vi "Durability_will_2012_07_09.vi"() -> ()   [LabVIEW 2011]
uses:
  <vilib>/DAQmx/read.llb/DAQmx Read (Analog 1D Wfm NChan NSamp).vi
  <vilib>/DAQmx/write.llb/DAQmx Write (Counter Time 1Chan 1Samp).vi
  <vilib>/measure/madcrms.llb/Basic Averaged DC-RMS for 1 Chan.vi
  <vilib>/DAQmx/miscellaneous.llb/DAQmx Fill In Error Info.vi
  <vilib>/Analysis/NI_AALBase.lvlib
  <vilib>/measure/NI_MAPro.lvlib
panel:
  in  "Motor1 ID":string
  in  "User":string
  in  "Comments (cleared when written to file)":string
  out "Motor 1 Elapsed Time (s)":string caption="Elapsed Time Text"
  out "Motor 1 Start Time":string caption="Start Time Text"
  out "Motor 1 Down":bool
  out "Long Write":bool caption="Time has Elapsed"
  out "Short Write":bool caption="Time has Elapsed"
  out "Temps":dynamicdata(graph) caption="Signal Out"
  out "Power Graph":dynamicdata(graph) caption="Collected Signals"
  out "Errors":errorcluster
  out "RPM":dynamicdata(graph) caption="Collected Signals"
  out "Motor RPM":dbl format="%#.0f"
  out "Motor Power (watts)":dbl format="%#.4f"
  out "Power to MC1 (watts)":dbl format="%#.4f"
  out "Voltage to MC1 (volts)":dbl format="%#.4f"
  out "Current to MC1  (amps)":dbl format="%#.4f"
  in  "Manual Start":bool
  in  "Power \nSetting":i8(slide) min=0 max=100 step=10 scale=0.0..100.0
  out "Motor Temp (F)":dbl format="%.1f"
  out "Tank Temp (F)":dbl format="%.1f"
  in  "Quit 4":bool
  out "Phase to Phase Voltage":waveform(dbl)(graph)
  out "Phase Current":waveform(dbl)(graph)
  # "Temperature"
  # "MC1"
  # "Motor Power and RPM"
  # "todo disable user and motor fields when file started writing"
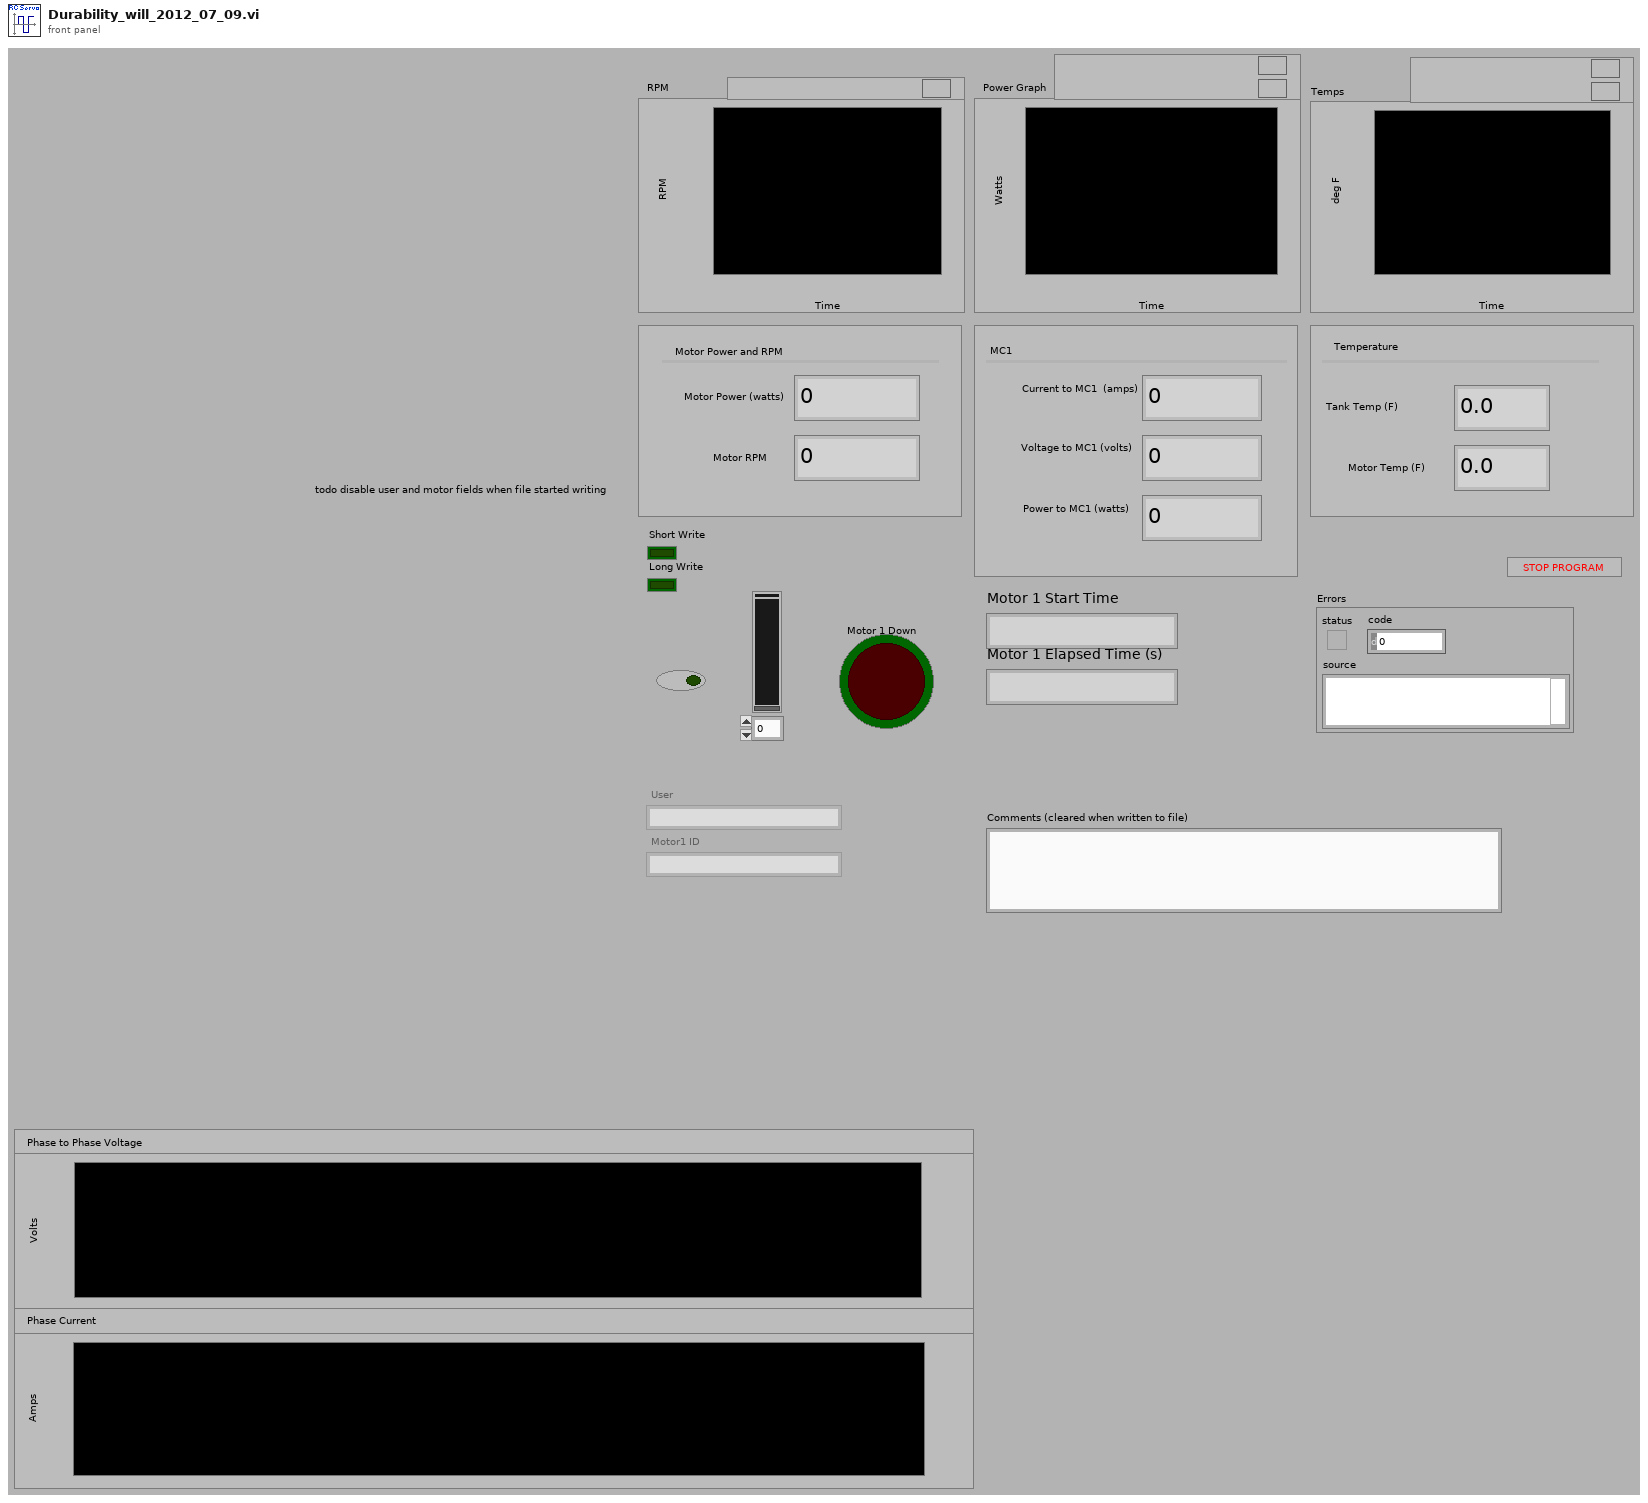
[diagram p1: front panel]
types:
  T1 = enum8{"Enabled", "Disabled", "Disabled and Grayed Out"}
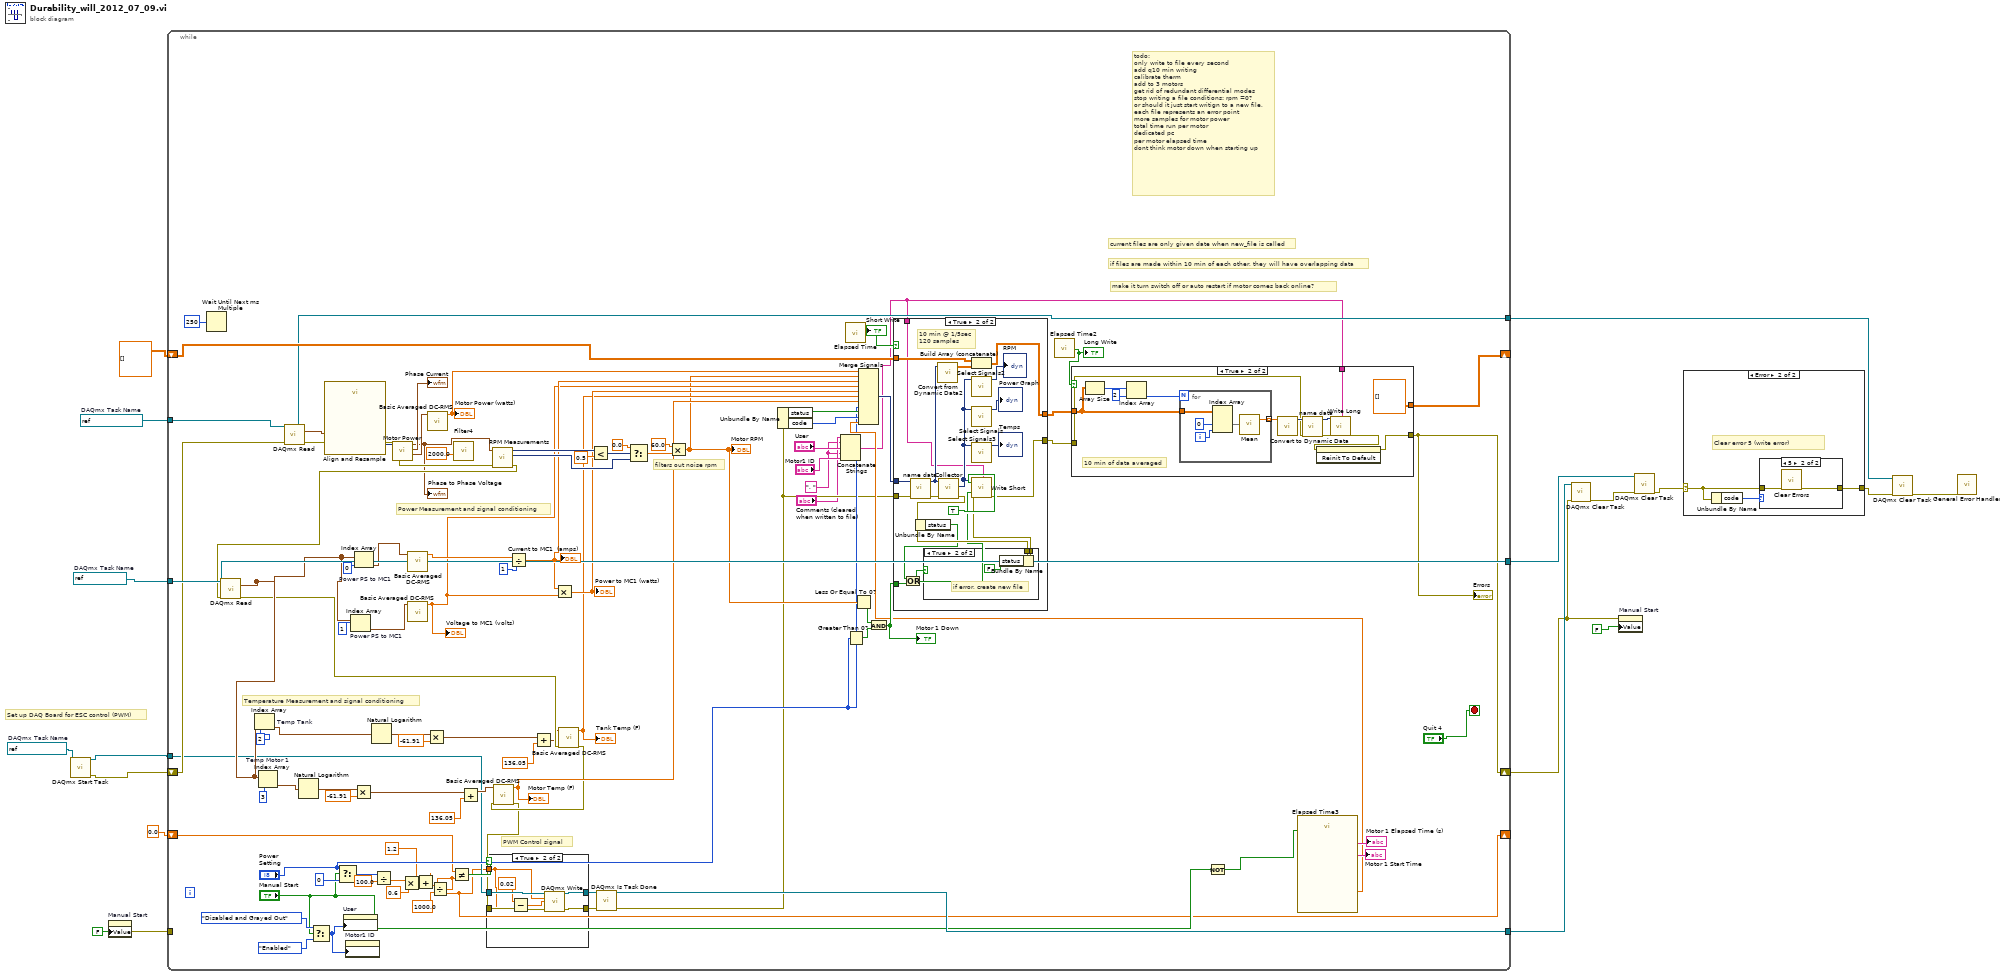
[diagram p0: block diagram]
diagram:
  w4 = refnum<k21> "PWM Signal"  # DAQmx Task Name
  w15 = refnum<k21> "MC Power"  # DAQmx Task Name
  w16 = refnum<k21> "Motor Power"  # DAQmx Task Name
  # "Set up DAQ Board for ESC control (PWM)"
  n1 = call <vilib>:"DAQmx Start Task.vi"("task/channels in"=w4) -> ("task out"=w3:refnum<k21>, "error out"=w2:errorcluster)  [unwired: 13 in]
  n2 = property on="Manual Start" class="Bool (strict)"("Value"=FALSE ("Run Motor")) -> (error out=w13:errorcluster)  [unwired: 2 in, 1 out]
  n3 = while {
    tunnel: [w115] -> w18
    tunnel: w3 -> [w38]
    shift-right: [w25] -> _
    shift-left: 0.0 -> [w40]
    tunnel: w15 -> [w107]
    tunnel: [w106] -> w17
    tunnel: [w57] -> w9
    tunnel: w16 -> [w96]
    tunnel: w13 -> [_]
    shift-right: [w60] -> _
    shift-left: dbl[][][] [] -> [w59]
    shift-right: [w32] -> w11
    shift-left: w2 -> [w54]
    stop <- "Quit 4" stop-if-true
    w20 = ", " ("string")
    # "PWM Control signal"
    # "make it turn switch off or auto restart if motor comes back online?"
    # "if files are made within 10 min of each other, they will have overlapping data"
    # "current files are only given date when new_file is called"
    # "todo:\nonly write to file every second\nadd q10 min writing\ncalibrate therm\nadd to 3 motors\nget rid of redundant differential modes\nstop writing a file conditions: rpm =0?\nor should it just start writign to a new file,\neach file represents an error point\nmore samples for motor power\ntotal time run per motor\ndedicated pc\nper motor elapsed time\ndont think motor down when starting up"
    # "filters out noise rpm"
    # "Power Measurement and signal conditioning"
    # "Temperature Measurement and signal conditioning"
    n4 = Wait Until Next ms Multiple(millisecond multiple=u32 250) -> ()  [unwired: 1 out]
    n5 = call-poly <vilib>:"DAQmx Read.vi"("task/channels in"=w96, "error in"=w54) -> ("task out"=w57:refnum<k21>, "data"=w79:waveform(dbl)[], "error out"=w55:errorcluster)  [unwired: 11 in]
    n6 = Select(t=T1."Disabled and Grayed Out" ("Disabled"), s="Manual Start", f=T1."Enabled" ("Disabled")) -> (s? t:f=w43:T1)
    n7 = call "Align and Resample"("Signals"=w79) -> ("Resampled Signals"=w80:dynamicdata)  [unwired: 8 in, 2 out]
    n8 = Select(t="Power \nSetting", s="Manual Start", f=i8 0) -> (s? t:f=w112:i8)
    n9 = property on="User" class="Str"("DisabledEnum"=w43) -> ()  [unwired: 2 in, 2 out]
    n10 = property on="Motor1 ID" class="Str"("DisabledEnum"=w43) -> ()  [unwired: 2 in, 2 out]
    n11 = Divide(x=w112, y=100.0) -> (x/y=w27:dbl)
    n12 = call "Motor Power.vi"("data"=w80) -> ("Waveform"=w74:waveform(dbl), "Phase Current"=→"Phase Current":waveform(dbl), "Phase to Phase Voltage"=w31:waveform(dbl))  [unwired: 7 in, 1 out]
    "Phase to Phase Voltage" <- w31
    n13 = Multiply(x=w27, y=0.6 ("scale")) -> (x*y=w24:dbl)
    n14 = Add(x=w24, y=1.2 ("add")) -> (x+y=w29:dbl)
    n15 = call-poly <vilib>:"Basic Averaged DC-RMS.vi"("signal in"=w74) -> ("DC value"=w73:dbl)  [unwired: 7 in, 3 out]
    "Motor Power (watts)" <- w73
    n16 = Divide(x=w29, y=1000.0) -> (x/y=w25:dbl)
    n17 = Not Equal?(x=w40, y=w25) -> (x != y?=w39:bool)
    n18 = call "Filter4"("Lower Cut-Off"=2000.0 ("LowPass Filter CutOff [Hz]")) -> ()  [unwired: 9 in, 2 out]
    n19 = call "RPM Measurements"("error in (no error)"=w55, "Signals"=w31) -> ("error out"=w95:errorcluster, "Frequency"=w101:dynamicdata, "Amplitude"=w98:dynamicdata)  [unwired: 7 in]
    n20 = call-poly <vilib>:"DAQmx Read.vi"("task/channels in"=w107, "error in"=w95) -> ("task out"=w106:refnum<k21>, "data"=w67:waveform(dbl)[], "error out"=w65:errorcluster)  [unwired: 11 in]
    n21 = Index Array "Temp Tank"(array=w67, index=2) -> (element=w68:waveform(dbl))
    n22 = Index Array "Temp Motor 1"(array=w67, index=3) -> (element=w90:waveform(dbl))
    n23 = Natural Logarithm(1:w90) -> (0:w94:waveform(dbl))
    n24 = Index Array "Power PS to MC1"(array=w67, index=1) -> (element=w70:waveform(dbl))
    n25 = Multiply(x=w94, y=-61.91) -> (x*y=w92:waveform(dbl))
    n26 = Index Array "Power PS to MC1"(array=w67, index=0) -> (element=w72:waveform(dbl))
    n27 = Natural Logarithm(1:w68) -> (0:w89:waveform(dbl))
    n28 = call-poly <vilib>:"Basic Averaged DC-RMS.vi"("signal in"=w72) -> ("DC value"=w71:dbl)  [unwired: 7 in, 3 out]
    n29 = call-poly <vilib>:"Basic Averaged DC-RMS.vi"("signal in"=w70) -> ("DC value"=w69:dbl)  [unwired: 7 in, 3 out]
    "Voltage to MC1 (volts)" <- w69
    n30 = Multiply(x=w89, y=-61.91) -> (x*y=w87:waveform(dbl))
    n31 = Add(x=w92, y=136.05) -> (x+y=w63:waveform(dbl))
    n32 = Divide(x=w71, y=1) -> (x/y=w84:dbl)
    "Current to MC1  (amps)" <- w84
    n33 = Add(x=w87, y=136.05) -> (x+y=w64:waveform(dbl))
    n34 = Multiply(x=w84, y=w69) -> (x*y=w83:dbl)
    "Power to MC1 (watts)" <- w83
    n35 = call-poly <vilib>:"Basic Averaged DC-RMS.vi"("error in (no error)"=w65, "signal in"=w64) -> ("error out"=w61:errorcluster, "DC value"=w66:dbl)  [unwired: 6 in, 2 out]
    "Tank Temp (F)" <- w66
    n36 = call-poly <vilib>:"Basic Averaged DC-RMS.vi"("error in (no error)"=w61, "signal in"=w63) -> ("error out"=w37:errorcluster, "DC value"=w62:dbl)  [unwired: 6 in, 2 out]
    "Motor Temp (F)" <- w62
    n37 = case shown="True" w39 {
      tunnel: [w117 w124] -> w36
      tunnel: [w116 w123] -> w35
      tunnel: w38 -> [w117 w122]
      tunnel: w37 -> [w116 w121]
      tunnel: w25 -> [_ w118]
      frame False {
      }
      frame True {
        n38 = Subtract(x=0.02 ("total time"), y=w118) -> (x-y=w120:dbl)
        n39 = call-poly <vilib>:"DAQmx Write.vi"("task/channels in"=w122, "high time"=w118, "low time"=w120, "error in"=w121) -> ("task out"=w124:refnum<k21>, "error out"=w123:errorcluster)  [unwired: 9 in, 1 out]
      }
    }
    n40 = Less?(x=w98, y=0.5) -> (x < y?=w100:dynamicdata)
    n41 = call <vilib>:"DAQmx Is Task Done.vi"("task/channels in"=w36, "error in"=w35) -> ("task out"=w115:refnum<k21>, "error out"=w34:errorcluster)  [unwired: 11 in, 1 out]
    n42 = Select(t=0.0, s=w100, f=w101) -> (s? t:f=w103:dbl)
    n43 = Multiply(x=60.0, y=w103) -> (x*y=w53:dbl)
    "Motor RPM" <- w53
    n44 = Unbundle By Name(w34) -> ("status"=w82:bool, "code"=w81:i32)
    n45 = Concatenate Strings("Comments (cleared when written to file)", w20, "User", w20, "Motor1 ID") -> (w19:string)
    n46 = call "Elapsed Time"() -> ("Time has Elapsed"=w77:bool)  [unwired: 12 in, 7 out]
    "Short Write" <- w77
    n47 = Greater Than 0?(x="Power \nSetting") -> (x > 0?=w51:bool)
    n48 = Less Or Equal To 0?(x=w53) -> (x <= 0?=w52:bool)
    n49 = And(x=w52, y=w51) -> (x .and. y?=w50:bool)
    "Motor 1 Down" <- w50
    n50 = call "Elapsed Time2"() -> ("Time has Elapsed"=w76:bool)  [unwired: 12 in, 7 out]
    "Long Write" <- w76
    n51 = Not(x="Manual Start") -> (.not. x?=w47:bool)
    n52 = call "Elapsed Time3"("Reset"=w47) -> ("Start Time Text"=→"Motor 1 Start Time":string, "Elapsed Time (s)"=w46:dbl, "Elapsed Time Text"=→"Motor 1 Elapsed Time (s)":string)  [unwired: 11 in, 5 out]
    n53 = Merge Signals(w73, w53, w84, w69, w83, w66, w62, "Power \nSetting", w82, w81, w46) -> (w75:dynamicdata)
    n54 = case shown="True" w77 {
      tunnel: w75 -> [_ w161]
      tunnel: w34 -> [w146 w158]
      tunnel: [w146 w153] -> w56
      tunnel: [w145 w165] -> w58
      tunnel: w59 -> [w145 w164]
      tunnel: w50 -> [_ w149]
      tunnel: w19 -> [_ w147]
      frame False {
      }
      frame True {
        # "10 min @ 1/5sec\n120 samples"
        n55 = call "name data.vi"("error in (no error)"=w158, "Dynamic Data"=w161) -> ("error out"=w159:errorcluster, "Output"=w160:dynamicdata)  [unwired: 8 in]
        n56 = call "Convert from Dynamic Data2"("Dynamic Data Type"=w160) -> ("Array"=w163:dbl[][])  [unwired: 3 in]
        n57 = call "Collector"("error in (no error)"=w159, "Signals"=w160) -> ("error out"=w151:errorcluster, "Collected Signals"=w154:dynamicdata)  [unwired: 8 in]
        n58 = Unbundle By Name(w151) -> ("status"=w150:bool)
        n59 = Or(x=w150, y=w149) -> (x .or. y?=w148:bool)
        n60 = case shown="True" w148 {
          tunnel: [w166 w169] -> w152
          tunnel: w151 -> [w166 w168]
          frame False {
          }
          frame True {
            # "if error, create new file"
            n61 = Bundle By Name(cluster=w168, "status"=FALSE) -> (w169:errorcluster)
          }
        }
        n62 = Build Array (concatenate)(w164, w163) -> (w165:dbl[][][])
        n63 = call "Select Signals2"("Signals"=w154) -> ("Signal Out"=→"RPM":dynamicdata)  [unwired: 9 in, 1 out]
        n64 = call "Select Signals"("Signals"=w154) -> ("Signal Out"=→"Power Graph":dynamicdata)  [unwired: 9 in, 1 out]
        n65 = call "Select Signals3"("Signals"=w154) -> ("Signal Out"=→"Temps":dynamicdata)  [unwired: 9 in, 1 out]
        n66 = call "Write Short"("Signals"=w154, "Reset"=TRUE, "new_file"=w148, "error in (no error)"=w152, "Comment"=w147) -> ("error out"=w153:errorcluster)  [unwired: 12 in, 2 out]
      }
    }
    n67 = case shown="True" w76 {
      tunnel: w58 -> [w126 w139]
      tunnel: [w126 dbl[][][] []] -> w60
      tunnel: w56 -> [w125 w131]
      tunnel: [w125 w127] -> w32
      tunnel: w19 -> [_ w129]
      frame False {
      }
      frame True {
        # "10 min of data averaged"
        n68 = Array Size(array=w139) -> (size(s)=w135:i32[])
        n69 = Index Array(array=w135, index=2) -> (element=w136:i32)
        n70 = for {
          N: w136 -> [_]
          tunnel: w139 -> [w144]
          tunnel: [w140] -> w134 mode=indexing
          i -> [w143]
          n71 = Index Array(array=w144, index (dim 1)=0 ("disabled index (row)"), index (dim 2)=w143) -> (element=w142:dbl[])  [unwired: 1 in]
          n72 = call <vilib>:"Mean.vi"("X"=w142) -> ("mean"=w140:dbl)  [unwired: 1 out]
        }
        n73 = call "Convert to Dynamic Data"("Array"=w134) -> ("Dynamic Data Type"=w133:dynamicdata)  [unwired: 3 in]
        n74 = call "name data.vi"("error in (no error)"=w131, "Dynamic Data"=w133) -> ("error out"=w130:errorcluster, "Output"=w132:dynamicdata)  [unwired: 8 in]
        n75 = call "Write Long"("Signals"=w132, "error in (no error)"=w130, "Comment"=w129) -> ("error out"=w128:errorcluster)  [unwired: 14 in, 2 out]
        n76 = invoke on="Comments (cleared when written to file)" class="Str" method="Reinit To Default"(error in=w128) -> (error out=w127:errorcluster)  [unwired: 2 in, 2 out]
      }
    }
    "Errors" <- w32
  }
  n77 = call <vilib>:"DAQmx Clear Task.vi"("task in"=w18, "error in"=w11) -> ("error out"=w5:errorcluster)  [unwired: 13 in]
  n78 = property on="Manual Start" class="Bool (strict)"(error in=w11, "Value"=FALSE ("Run Motor")) -> ()  [unwired: 1 in, 2 out]
  n79 = call <vilib>:"DAQmx Clear Task.vi"("task in"=w17, "error in"=w5) -> ("error out"=w7:errorcluster)  [unwired: 13 in]
  n80 = case shown="Error" w7 {
    selector: w7 -> [w170 w172]
    tunnel: [w170 w171] -> w6
    frame No Error {
    }
    frame Error {
      # "Clear error 5 (write error)"
      n81 = Unbundle By Name(w172) -> ("code"=w173:i32)
      n82 = case shown="5" w173 {
        tunnel: w172 -> [w174 w176]
        tunnel: [w174 w175] -> w171
        frame Default {
        }
        frame 5 {
          n83 = call <vilib>:"Clear Errors.vi"("error in (no error)"=w176) -> ("error out"=w175:errorcluster)  [unwired: 6 in]
        }
      }
    }
  }
  n84 = call <vilib>:"DAQmx Clear Task.vi"("task in"=w9, "error in"=w6) -> ("error out"=w8:errorcluster)  [unwired: 13 in]
  n85 = call <vilib>:"General Error Handler.vi"("error in (no error)"=w8) -> ()  [unwired: 10 in, 5 out]
